vi "DHT11 (FPGA).vi"() -> ()   [LabVIEW 2015, in "DHT11 (FPGA).lvlib"]
uses:
  DHT11 (FPGA).lvlib
  <vilib>/rvi/Emulation/niFpgaGetClockAttributes.vi
  <vilib>/rvi/Emulation/niFpgaSctlEmulationGetInTimedLoop.vi
  <vilib>/rvi/Emulation/niFpgaEmulationReportErrorSimple.vi
  <vilib>/rvi/Emulation/niFpgaCriticalErrorInLSC.vi
panel:
  out "Temperature (°C)":u8
  out "Humidity (%)":u8
  out "error out":errorcluster
  in  "Loop Rate in ms (1000)":u32=1000 min=2000
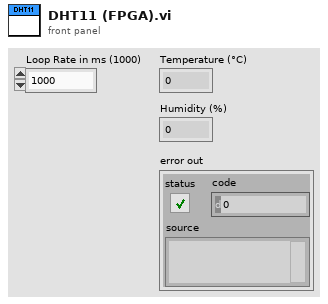
[diagram p1: front panel]
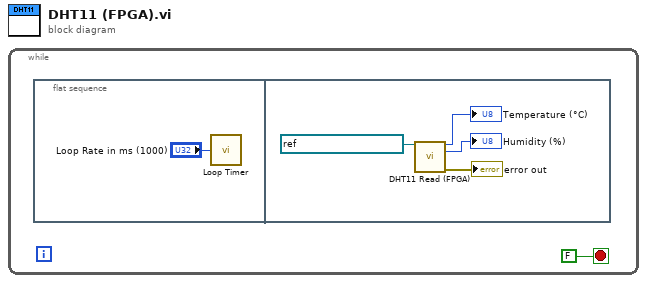
[diagram p0: block diagram]
diagram:
  n1 = while {
    stop <- FALSE stop-if-true
    n2 = flat-sequence {
      frame #0 {
        n3 = call "Loop Timer"("Count(mSec)"="Loop Rate in ms (1000)") -> ()  [unwired: 1 out]
      }
      frame #1 {
        n4 = call "DHT11 Read (FPGA).vi"("FPGA I/O In"=refnum<k21> "ConnectorA/DIO0") -> ("Temperature (°C)"=→"Temperature (°C)":u8, "Humidity (%)"=→"Humidity (%)":u8, "error out"=→"error out":errorcluster)  [unwired: 12 in]
      }
    }
  }
